vi "Open Project.vi"(8 "error in (no error)":errorcluster, 11 "PostBuildSupport in":refnum<class "PostBuildSupport.lvclass">) -> (0 "error out":errorcluster, 3 "PostBuildSupport out":refnum<class "PostBuildSupport.lvclass">)   [LabVIEW 2019, in "PostBuildSupport.lvclass"]
uses:
  PostBuildSupport.lvclass
  Build/Typedefs/Build Spec Type--combo.ctl
  PostBuildSupport.lvclass/PostBuildSupport.ctl
  Build/Build.lvlib
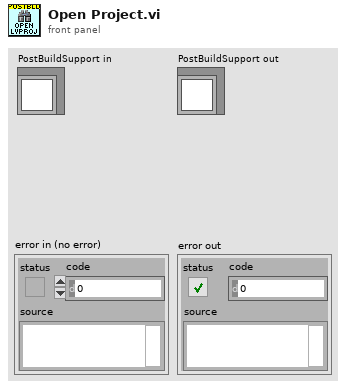
[diagram p1: front panel]
types:
  T1 = typedef "Build.lvlib/Build Spec Type--combo.ctl" = string
  T2 = typedef "Build.lvlib/Build Spec--cluster.ctl" = cluster{"Name":string, "Type":string, "Version":string}
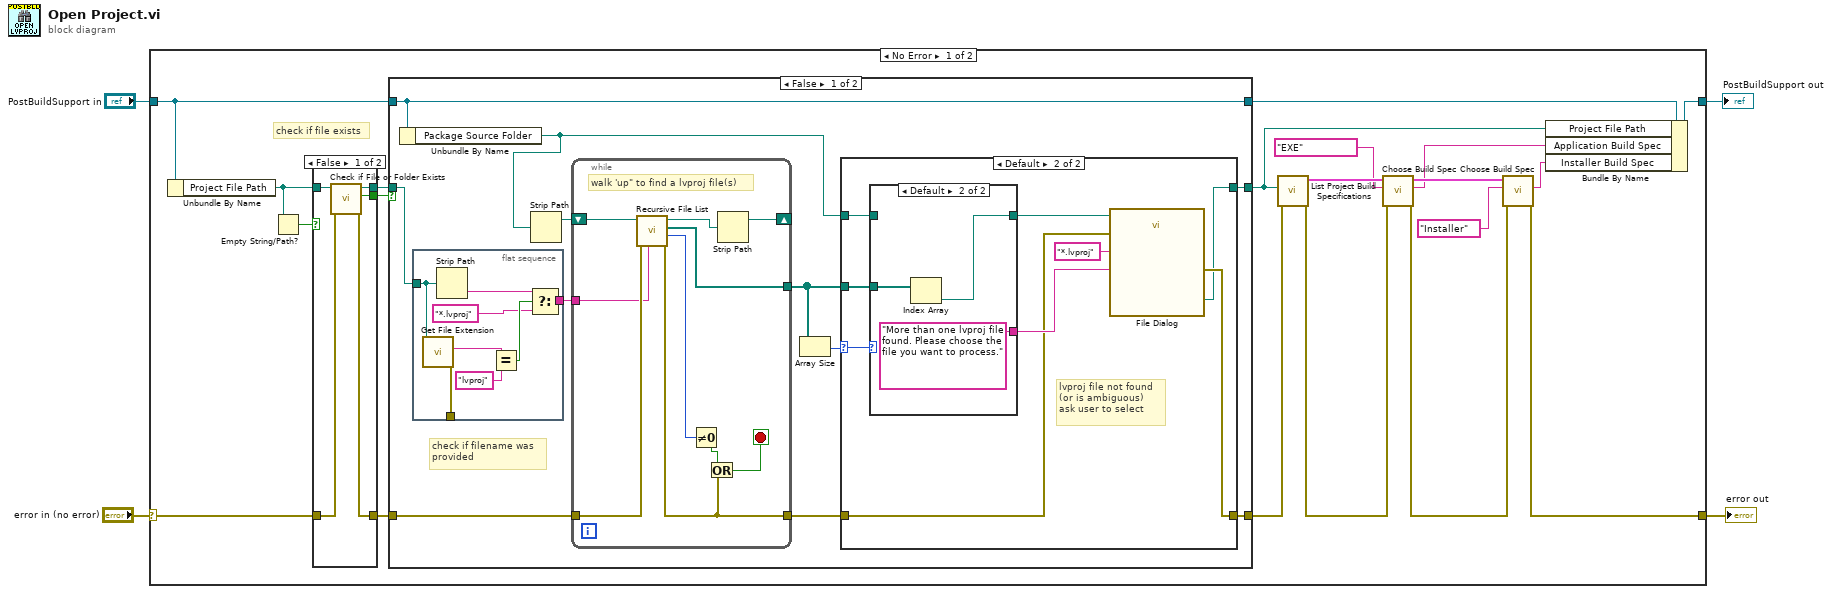
[diagram p0: block diagram]
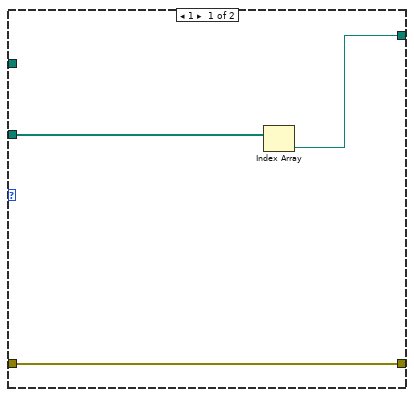
[diagram p2: hidden frame]
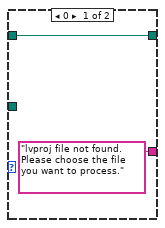
[diagram p3: hidden frame]
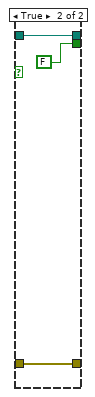
[diagram p5: hidden frame]
diagram:
  n1 = case shown="No Error" "error in (no error)" {
    selector: "error in (no error)" -> [w18 w83]
    tunnel: "PostBuildSupport in" -> [w19 w82]
    tunnel: [w7 w83] -> w2
    tunnel: [w24 w82] -> w1
    frame No Error {
      # "check if file exists"
      n2 = Unbundle By Name(w19) -> ("Project File Path"=w6:path)
      n3 = Empty String/Path?(string/path=w6) -> (empty?=w12:bool)
      n4 = case shown="False" w12 {
        tunnel: w18 -> [w78 w80]
        tunnel: [w77 w80] -> w17
        tunnel: [w76 FALSE ("file or folder exists?")] -> w16
        tunnel: [w75 w79] -> w15
        tunnel: w6 -> [w74 w79]
        frame False {
          n5 = call <vilib>:"Check if File or Folder Exists.vi"("error in (no error)"=w78, "path"=w74) -> ("error out"=w77:errorcluster, "file or folder exists?"=w76:bool, "dup path"=w75:path)  [unwired: 7 in]
        }
        frame True {
        }
      }
      n6 = case shown="False" w16 {
        tunnel: [w32 w73] -> w5
        tunnel: w19 -> [w30 w72]
        tunnel: w17 -> [w31 w71]
        tunnel: w15 -> [w25 w73]
        tunnel: [w30 w72] -> w14
        tunnel: [w28 w71] -> w13
        frame False {
          # "check if filename was\nprovided"
          n7 = Unbundle By Name(w30) -> ("Package Source Folder"=w27:path)
          n8 = flat-sequence {
            tunnel: [w43] -> w26
            tunnel: w25 -> [w37]
            tunnel: [w36] -> _
            frame #0 {
              n9 = call <vilib>:"Get File Extension.vi"("file"=w37) -> ("error out"=w36:errorcluster, "lowercase file extension"=w42:string)  [unwired: 6 in, 3 out]
              n10 = Strip Path(path=w37) -> (name=w39:string)  [unwired: 1 out]
              n11 = Equal?(x=w42, y="lvproj" ("pattern")) -> (x = y?=w40:bool)
              n12 = Select(t=w39, s=w40, f="*.lvproj" ("pattern")) -> (s? t:f=w43:string)
            }
          }
          n13 = Strip Path(path=w27) -> (stripped path=w35:path)  [unwired: 1 out]
          n14 = while {
            tunnel: [w65] -> w29
            tunnel: w31 -> [w67]
            shift-right: [w69] -> _
            shift-left: w35 -> [w66]
            tunnel: [w62] -> w33
            tunnel: w26 -> [w61]
            stop <- w63 stop-if-true
            # "walk 'up\" to find a lvproj file(s)"
            n15 = call <vilib>:"Recursive File List.vi"("pattern"=w61, "error in (no error)"=w67, "Folder Path"=w66) -> ("error out"=w65:errorcluster, "Number of Files"=w70:i32, "All Files in Dir"=w62:path[], "dup Folder Path"=w68:path)  [unwired: 4 in, 1 out]
            n16 = Not Equal To 0?(x=w70) -> (x != 0?=w64:bool)
            n17 = Or(x=w64, y=w65) -> (x .or. y?=w63:bool)
            n18 = Strip Path(path=w68) -> (stripped path=w69:path)  [unwired: 1 out]
          }
          n19 = Array Size(array=w33) -> (size(s)=w34:i32)
          n20 = case shown="Default" w34 {
            selector: w34 -> [_ w54]
            tunnel: w33 -> [w46 w53]
            tunnel: [w45 w47] -> w32
            tunnel: w27 -> [_ w50]
            tunnel: w29 -> [w44 w49]
            tunnel: [w44 w48] -> w28
            frame 1 {
              n21 = Index Array(array=w46) -> (element=w45:path)  [unwired: 1 in]
            }
            frame Default {
              # "lvproj file not found\n(or is ambiguous)\nask user to select"
              n22 = case shown="Default" w54 {
                tunnel: w53 -> [_ w60]
                tunnel: [w56 w59] -> w52
                tunnel: ["lvproj file not found. Please choose the file you want to process." ("prompt") "More than one lvproj file found. Please choose the file you want to process." ("prompt")] -> w51
                tunnel: w50 -> [w56 _]
                frame 0 {
                }
                frame Default {
                  n23 = Index Array(array=w60) -> (element=w59:path)  [unwired: 1 in]
                }
              }
              n24 = call "File Dialog"("start path"=w52, "prompt"=w51, "error in"=w49, "pattern label"="*.lvproj") -> ("selected path"=w47:path, "error out"=w48:errorcluster)  [unwired: 8 in, 2 out]
            }
          }
        }
        frame True {
        }
      }
      n25 = call "List Project Build Specifications.vi"("error in (no error)"=w13, "project path"=w5) -> ("error out"=w8:errorcluster, "Build Specs"=w23:T2[])  [unwired: 8 in]
      n26 = call "Choose Build Spec.vi"("error in"=w8, "Build Type"=T1 "EXE", "Build Specs"=w23) -> ("error out"=w11:errorcluster, "Name"=w10:string, "Build Specs out"=w22:T2[])  [unwired: 5 in, 1 out]
      n27 = call "Choose Build Spec.vi"("error in"=w11, "Build Type"=T1 "Installer", "Build Specs"=w22) -> ("error out"=w7:errorcluster, "Name"=w9:string)  [unwired: 5 in, 2 out]
      n28 = Bundle By Name(cluster=w14, "Project File Path"=w5, "Application Build Spec"=w10, "Installer Build Spec"=w9) -> (w24:refnum<class "PostBuildSupport.lvclass">)
    }
    frame Error {
    }
  }
  "error out" <- w2
  "PostBuildSupport out" <- w1
